vi "[RE Python] Parse Elf Claims.vi"(8 "error in (no error)":errorcluster, 11 "1D String Array":string[](array[string])) -> (0 "Error Out":errorcluster, 3 "Elf Claims":string[][](array[string]))   [LabVIEW 2019]
doc: "Given a 1D string array of strings in the format \"#<claim ID> @ <distance from top edge>,<distance from left edge>: <width>x<height>\" or an actual example \"#1 @ 1,3: 4x4\", parse each of the numbers out into its own row."
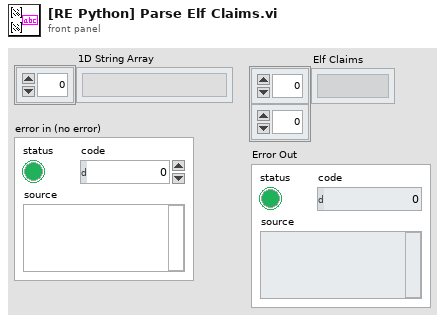
[diagram p1: front panel]
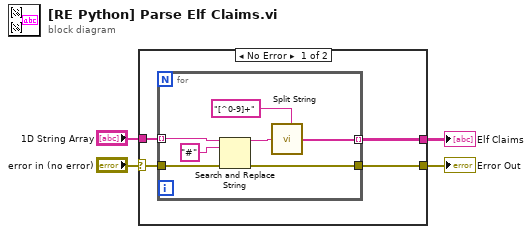
[diagram p0: block diagram]
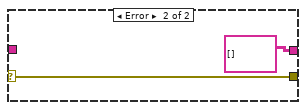
[diagram p2: hidden frame]
diagram:
  n1 = case shown="No Error" "error in (no error)" {
    selector: "error in (no error)" -> [w6 w17]
    tunnel: [w8 string[][] [] ("Split String")] -> w4
    tunnel: "1D String Array" -> [w7 _]
    tunnel: [w5 w17] -> w1
    frame No Error {
      n2 = for {
        tunnel: w7 -> [w12] mode=indexing
        tunnel: w6 -> [w11]
        tunnel: [w10] -> w8 mode=indexing
        tunnel: [w9] -> w5
        n3 = Search and Replace String(input string=w12, search string="#", error in=w11) -> (result string=w13:string, error out=w9:errorcluster)  [unwired: 5 in, 2 out]
        n4 = call <vilib>:"Split String.vi"("Split Pattern"="[^0-9]+", "Input String"=w13) -> ("Split String"=w10:string[])  [unwired: 5 in]
      }
    }
    frame Error {
    }
  }
  "Elf Claims" <- w4
  "Error Out" <- w1
